vi "Connect.vi"(8 "error in (no error)":errorcluster, 10 "Addon Name":string, 11 "Address":string) -> (0 "error out":errorcluster, 3 "Ref":T1)   [LabVIEW 2019, in "Ghost Bus Host Automation API.lvlib"]
uses:
  Ghost Bus Host Automation API.lvlib
  <vilib>/NI/STM/NI STM.lvlib
  <vilib>/NI/STM/TCP/Write Meta Data (TCP Ref).vi
  <vilib>/NI/STM/SubVIs/MetaDataElement.ctl
  <vilib>/NI/STM/TCP/TCP Connection Info.ctl
  Types/API Variables.ctl
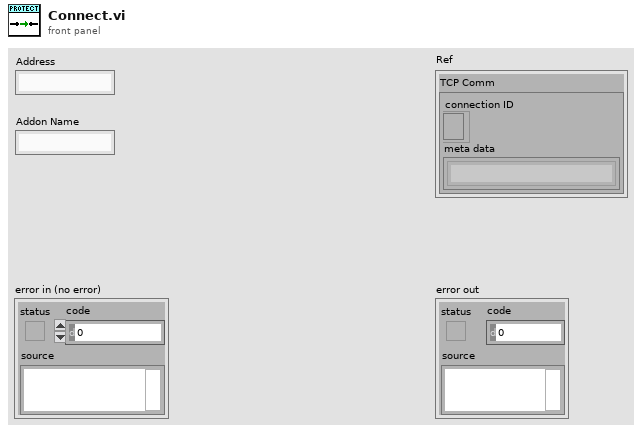
[diagram p1: front panel]
types:
  T1 = typedef "Ghost Bus Host Automation API.lvlib/API Variables.ctl" = cluster{"TCP Comm":T2}
  T2 = typedef "NI STM.lvlib/TCP Connection Info.ctl" = cluster{"connection ID":refnum<k5>, "meta data":T3[]}
  T3 = typedef "NI STM.lvlib/MetaDataElement.ctl" = string
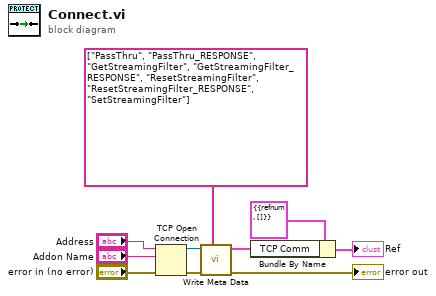
[diagram p0: block diagram]
diagram:
  n1 = TCP Open Connection(address="Address", remote port or service name="Addon Name", error in (no error)="error in (no error)") -> (connection ID=w9:refnum<k5>, error out=w10:errorcluster)  [unwired: 2 in]
  n2 = call-poly <vilib>:"Write Meta Data.vi"("meta data"=string[] ["PassThru", "PassThru_RESPONSE", "GetStreamingFilter", "GetStreamingFilter_RESPONSE", "ResetStreamingFilter", "ResetStreamingFilter_RESPONSE", "SetStreamingFilter"] ("Meta data"), "error in"=w10, "connection ID"=w9) -> ("error out"=→"error out":errorcluster, "connection info out"=w2:T2)  [unwired: 7 in]
  n3 = Bundle By Name(cluster=T1 {"TCP Comm"={"connection ID"=refnum, "meta data"=[]}} ("Ref 2"), "TCP Comm"=w2) -> (→"Ref":T1)
